vi "UseFGV3.vi"() -> ()   [LabVIEW 2019]
panel:
  in  "stop":bool
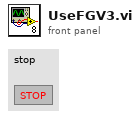
[diagram p1: front panel]
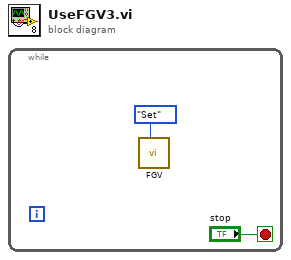
[diagram p0: block diagram]
diagram:
  n1 = while {
    stop <- "stop" stop-if-true
    n2 = call "FGV.vi"("State"=enum16{"Set", "Get"}."Set") -> ()  [unwired: 10 in, 1 out]
  }
